vi "Handle Error.vi"(8 "error in (no error)":errorcluster, 11 "VG-VNA_GUI in":refnum<class "VG-VNA_GUI.lvclass">) -> (0 "error out":errorcluster, 2 "stop actor?":bool=TRUE, 3 "VG-VNA_GUI out":refnum<class "VG-VNA_GUI.lvclass">)   [LabVIEW 2020, in "VG-VNA_GUI.lvlib" / "VG-VNA_GUI.lvclass"]
doc: "(<B>Filename</B>: Actor Framework.lvlib:Actor.lvclass:Handle Error.vi)\n\nDefines how the actor handles an error that occurred while processing a message. By default, this method does nothing except stop the actor."
uses:
  VG-VNA_GUI.lvclass
  <vilib>/ActorFramework/Actor/Actor.lvclass
  common/features/CF-common_features.lvlib
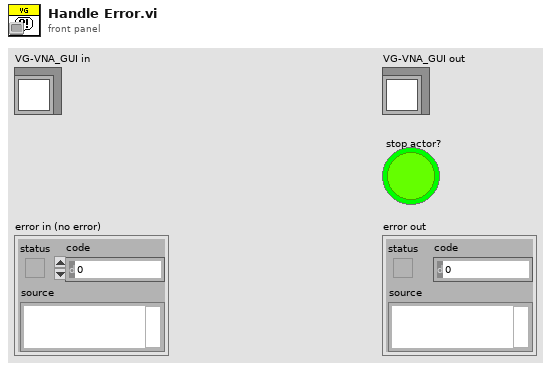
[diagram p1: front panel]
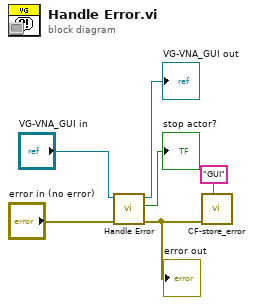
[diagram p0: block diagram]
diagram:
  n1 = call-parent "Handle Error.vi"("error in (no error)"="error in (no error)", "Actor in"="VG-VNA_GUI in") -> ("error out"=w2:errorcluster, "stop actor?"=→"stop actor?":bool, "Actor out"=→"VG-VNA_GUI out":refnum<class "VG-VNA_GUI.lvclass">)  [unwired: 7 in]
  "error out" <- w2
  n2 = call "CF-store_error.vi"("Location"="GUI", "error in (no error)"=w2) -> ()  [unwired: 10 in]
